vi "Y_switch_control.vi"(9 "Y":T2={"Y_HSw"=0, "Y_HSetState"=enum."hand", "Y_ASetState"=enum."hand", "Y_DSetState"=enum."hand"} {"Y_HSw" max=2 step=1}, 10 "Z_State":T1=enum."disabled", 11 "Y_LSw (2-auto)":u32=2) -> (2 "Y_SetState":T3=enum."hand", 3 "Y_Source":T4=enum."local hand")   [LabVIEW 2019, in "control.lvlib"]
doc: "Y_Source – источник выхода\n 0 – initialize (Инициализация)\n 1 – local disabled (Выведен из работы по месту)\n 2 – local hand (Ручной местный)\n 3 – hand (Ручной контроллера)\n 4 – auto (Автомат контроллера)\n 5 – dist (Дистанционный)\nY_SetState заданное состояние выхода:\n 0 – initialize (Инициализация) \n 1 – alarm (Аварийное значение)\n 2 – min (Минимальное значение)\n 3 – stop (Остановлен)\n 4 – forced (Принудительное (ручное) задание)\n 5 – auto (Автомат (ПИД регулятор))\n 6 – max (Максимум)"
uses:
  control.lvlib
  ctl/Y_source.ctl
  ctl/Y_state.ctl
  ctl/Y_control.ctl
  ctl/Z_State.ctl
  Heating/ctl/Y_state.ctl
  Heating/Heating.lvlib
panel:
  # "Входы\nY_LSw – переключатель р/а. 1 приоритет\n     0 – откл\n     1 – ручной (местный)\n     2 – автомат\nY_HSw – источник выхода из меню. 2 приоритет\n     0 – ручной контроллера\n     1 – автомат контроллера\n     2 – дистационный\nY_HSetState – заданное состояние в меню или на панели\nY_ASetState – автоматически заданное состояние от вышестоящего алгоритма\nY_DSetState – дистанционно заданное состояние\n     ..0 – initialize (Инициализация)  -> 4 – автомат \n     1 – alarm (Аварийное значение)\n     2 – min (Минимальное значение)\n     3 – stop (Остановлен)\n     4 – forced (Принудительное (ручное) задание)\n     5 – auto (Автомат (ПИД регулятор))\n     6 – max (Максимум)\n     7.. -> 4 – автомат"
  # "Выходы\nY_Source – источник выхода\n     0 – initialize (Инициализация)\n     1 – local disabled (Выведен из работы по месту)\n     2 – local hand (Ручной местный)\n     3 – hand (Ручной контроллера)\n     4 – auto (Автомат контроллера)\n     5 – dist (Дистанционный)\nY_SetState заданное состояние выхода:\n     0 – initialize (Инициализация) \n     1 – alarm (Аварийное значение)\n     2 – min (Минимальное значение)\n     3 – stop (Остановлен)\n     4 – forced (Принудительное (ручное) задание)\n     5 – auto (Автомат (ПИД регулятор))\n     6 – max (Максимум)"
  # "Z_State(Z3) состояние автомата механизма:\n     0 – initialise (инициализация)\n     1 – alarm (авария)\n     2 – disabled (выведен из работы)\n     3 – not ready (не готов к работе)\n     4 – stop (стоп - готов к работе)\n     5 – reserv (резерв)\n     6 – switched off (отключается)\n     8 – switched on (включается)\n     9 – check (проверка работоспособности)\n     10 – on min (включен на минимуме)\n     11 – increase out (увеличение рабочего параметра)\n     12 – on (включен)\n     13 – decrease out (уменьшение рабочего параметра)\n     14 – on max (включен на максимуме)"
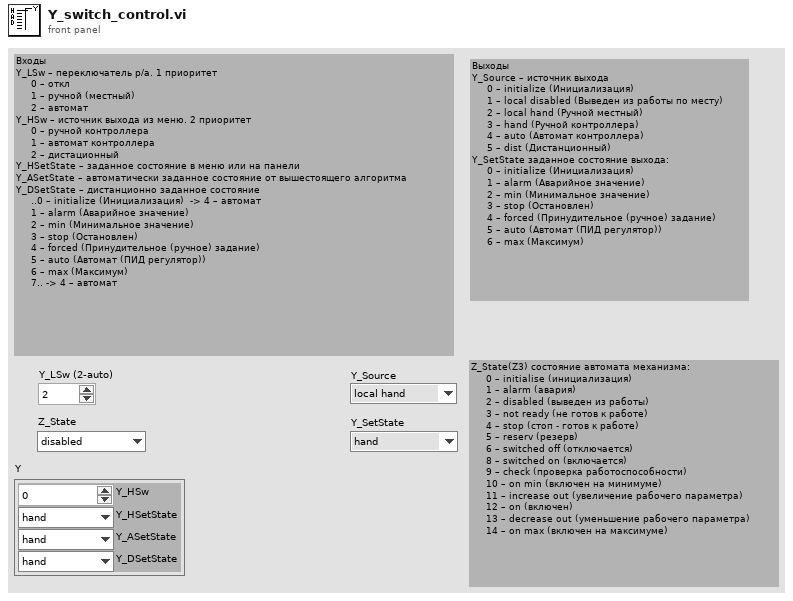
[diagram p1: front panel]
types:
  T1 = typedef "control.lvlib/Z_State.ctl" = enum8{"initialization", "alarm", "disabled", "not ready", "stop ready", "reserv", "switched off", "reserv2", "switched on", "check", "on min", "decrease out", "on", "increase out", "on max"}
  T2 = typedef "control.lvlib/Y_control.ctl" = cluster{"Y_HSw":u32, "Y_HSetState":T3, "Y_ASetState":T3, "Y_DSetState":T3}
  T3 = typedef "control.lvlib/Y_state.ctl" = enum8{"initialize", "alarm", "min", "stop", "hand", "auto", "max"}
  T4 = typedef "control.lvlib/Y_source.ctl" = enum8{"initialize", "local disabled", "local hand", "hand", "auto", "dist"}
  T5 = typedef "Heating.lvlib/Y_state.ctl" = enum8{"initialize", "alarm", "min", "stop", "hand", "auto", "max"}
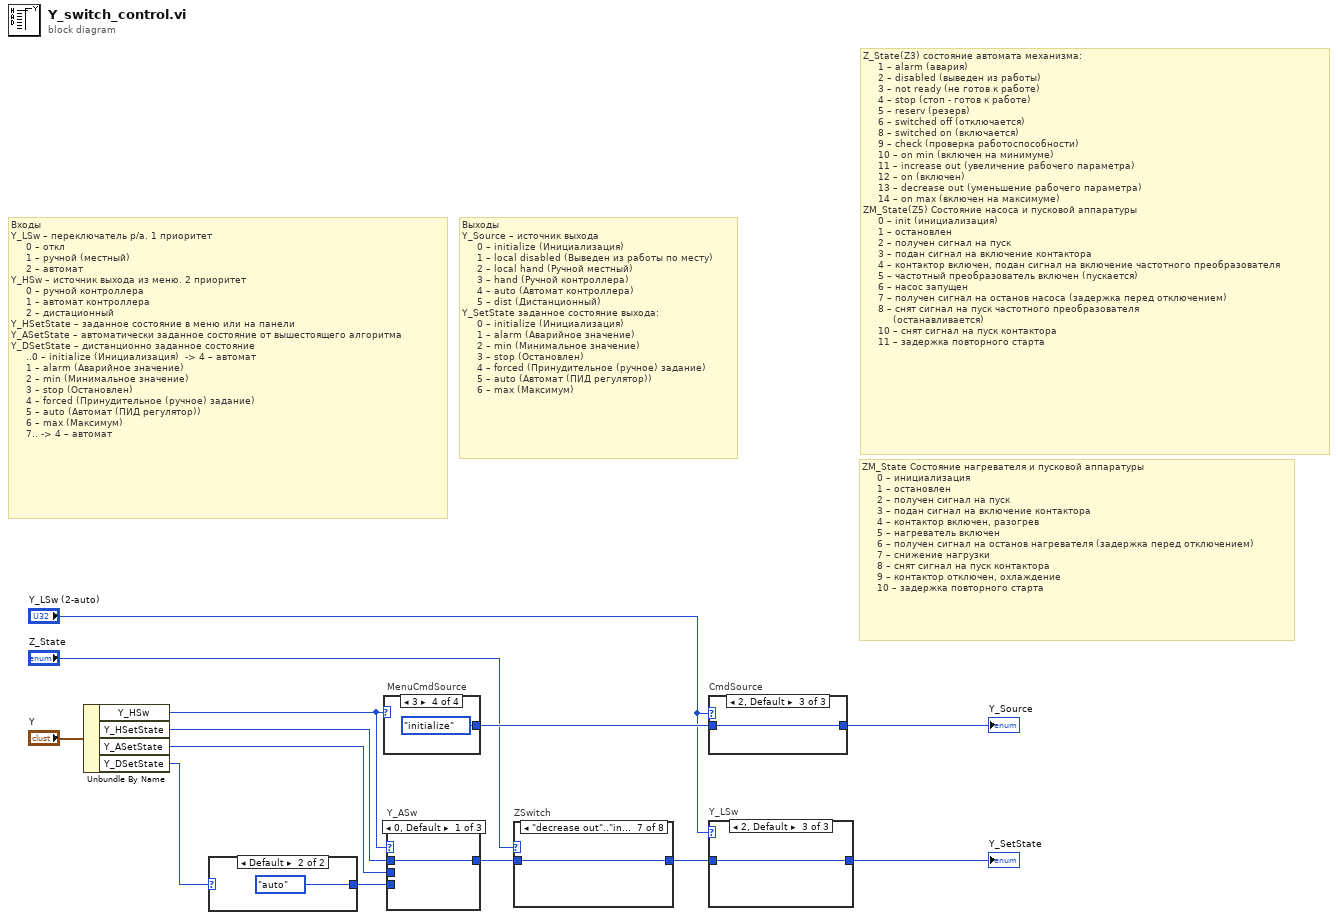
[diagram p0: block diagram]
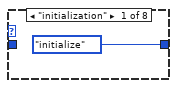
[diagram p2: hidden frame]
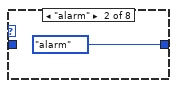
[diagram p3: hidden frame]
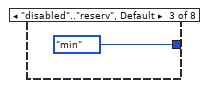
[diagram p4: hidden frame]
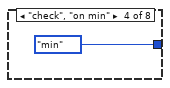
[diagram p5: hidden frame]
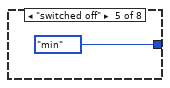
[diagram p6: hidden frame]
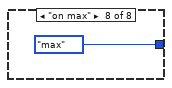
[diagram p8: hidden frame]
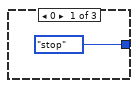
[diagram p12: hidden frame]
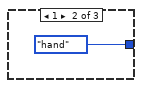
[diagram p13: hidden frame]
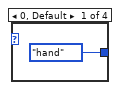
[diagram p14: hidden frame]
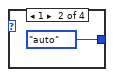
[diagram p15: hidden frame]
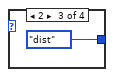
[diagram p16: hidden frame]
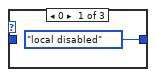
[diagram p17: hidden frame]
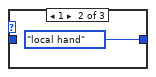
[diagram p18: hidden frame]
diagram:
  # "ZM_State Состояние нагревателя и пусковой аппаратуры\n     0 – инициализация\n     1 – остановлен\n     2 – получен сигнал на пуск\n     3 – подан сигнал на включение контактора\n     4 – контактор включен, разогрев\n     5 – нагреватель включен\n     6 – получен сигнал на останов нагревателя (задержка перед отключением)\n     7 – снижение нагрузки\n     8 – снят сигнал на пуск контактора\n     9 – контактор отключен, охлаждение\n     10 – задержка повторного старта"
  # "Z_State(Z3) состояние автомата механизма:\n     1 – alarm (авария)\n     2 – disabled (выведен из работы)\n     3 – not ready (не готов к работе)\n     4 – stop (стоп - готов к работе)\n     5 – reserv (резерв)\n     6 – switched off (отключается)\n     8 – switched on (включается)\n     9 – check (проверка работоспособности)\n     10 – on min (включен на минимуме)\n     11 – increase out (увеличение рабочего параметра)\n     12 – on (включен)\n     13 – decrease out (уменьшение рабочего параметра)\n     14 – on max (включен на максимуме)\nZM_State(Z5) Состояние насоса и пусковой аппаратуры\n     0 – init (инициализация)\n     1 – остановлен\n     2 – получен сигнал на пуск\n     3 – подан сигнал на включение контактора\n     4 – контактор включен, подан сигнал на включение частотного преобразователя\n     5 – частотный преобразователь включен (пускается)\n     6 – насос запущен\n     7 – получен сигнал на останов насоса (задержка перед отключением)\n     8 – снят сигнал на пуск частотного преобразователя\n          (останавливается)\n     10 – снят сигнал на пуск контактора\n     11 – задержка повторного старта"
  # "Входы\nY_LSw – переключатель р/а. 1 приоритет\n     0 – откл\n     1 – ручной (местный)\n     2 – автомат\nY_HSw – источник выхода из меню. 2 приоритет\n     0 – ручной контроллера\n     1 – автомат контроллера\n     2 – дистационный\nY_HSetState – заданное состояние в меню или на панели\nY_ASetState – автоматически заданное состояние от вышестоящего алгоритма\nY_DSetState – дистанционно заданное состояние\n     ..0 – initialize (Инициализация)  -> 4 – автомат \n     1 – alarm (Аварийное значение)\n     2 – min (Минимальное значение)\n     3 – stop (Остановлен)\n     4 – forced (Принудительное (ручное) задание)\n     5 – auto (Автомат (ПИД регулятор))\n     6 – max (Максимум)\n     7.. -> 4 – автомат"
  # "Выходы\nY_Source – источник выхода\n     0 – initialize (Инициализация)\n     1 – local disabled (Выведен из работы по месту)\n     2 – local hand (Ручной местный)\n     3 – hand (Ручной контроллера)\n     4 – auto (Автомат контроллера)\n     5 – dist (Дистанционный)\nY_SetState заданное состояние выхода:\n     0 – initialize (Инициализация) \n     1 – alarm (Аварийное значение)\n     2 – min (Минимальное значение)\n     3 – stop (Остановлен)\n     4 – forced (Принудительное (ручное) задание)\n     5 – auto (Автомат (ПИД регулятор))\n     6 – max (Максимум)"
  n1 = Unbundle By Name("Y") -> ("Y_HSw"=w6:u32, "Y_HSetState"=w5:T3, "Y_ASetState"=w4:T3, "Y_DSetState"=w3:T3)
  n2 = case shown="Default" w3 {
    selector: w3 -> [w14 _]
    tunnel: [w14 Y_state."auto" ("X1(SetState)")] -> w11
    frame "alarm".."max" {
    }
    frame Default {
    }
  }
  n3 = case "MenuCmdSource" shown="3" w6 {
    tunnel: [Y_source."hand" ("Z1(CmdSource) 3") Y_source."auto" ("Z1(CmdSource) 3") Y_source."dist" ("Z1(CmdSource) 3") Y_source."initialize" ("Z1(CmdSource) 3")] -> w13
    frame 0, Default {
    }
    frame 1 {
    }
    frame 2 {
    }
    frame 3 {
    }
  }
  n4 = case "Y_ASw" shown="0, Default" w6 {
    tunnel: [w20 w21 w22] -> w9
    tunnel: w5 -> [w20 _ _]
    tunnel: w11 -> [_ _ w22]
    tunnel: w4 -> [_ w21 _]
    frame 0, Default {
    }
    frame 1 {
    }
    frame 2 {
    }
  }
  n5 = case "ZSwitch" shown="\"decrease out\"..\"increase out\"" "Z_State" {
    tunnel: [Y_state."initialize" ("Y_HSetState") Y_state."alarm" ("Y_HSetState") Y_state."min" ("Y_HSetState") Y_state."min" ("Y_HSetState") Y_state."min" ("Y_HSetState") w28 w29 Y_state."max" ("Y_HSetState")] -> w8
    tunnel: w9 -> [_ _ _ _ _ w28 w29 _]
    frame "initialization" {
    }
    frame "alarm" {
    }
    frame "disabled".."reserv", Default {
    }
    frame "check", "on min" {
    }
    frame "switched off" {
    }
    frame "switched on" {
    }
    frame "decrease out".."increase out" {
    }
    frame "on max" {
    }
  }
  n6 = case "CmdSource" shown="2, Default" "Y_LSw (2-auto)" {
    tunnel: [Y_source."local disabled" ("Z1(CmdSource) 3") Y_source."local hand" ("Z1(CmdSource) 3") w33] -> w1
    tunnel: w13 -> [_ _ w33]
    frame 0 {
    }
    frame 1 {
    }
    frame 2, Default {
    }
  }
  "Y_Source" <- w1
  n7 = case "Y_LSw" shown="2, Default" "Y_LSw (2-auto)" {
    tunnel: [Y_state."stop" ("X1(SetState)") Y_state."hand" ("X1(SetState)") w36] -> w10
    tunnel: w8 -> [_ _ w36]
    frame 0 {
    }
    frame 1 {
    }
    frame 2, Default {
    }
  }
  "Y_SetState" <- w10
